vi "Configure lbd for pow meas.vi"(8 "error in (no error)":errorcluster, 10 "Meas lbd (span 0.1 nm)":dbl=895.0 format="%#.6g", 11 "VISA resource name":refnum<visa-resource-name>) -> (0 "error out":errorcluster, 3 "VISA resource name out":refnum<visa-resource-name>)   [LabVIEW 2021, in "Ceyear.lvlib"]
doc: "Configures the frequency range of the spectrum analyzer using the center frequency and the frequency span. If span corresponds to zero Hertz, then the spectrum analyzer operates in time-domain mode. Otherwise, spectrum analyzer operates in frequency-domain mode.\n\n Frequency Start = Center Frequency - Span/2\n Frequency Stop = Center Frequency + Span/2"
uses:
  <instrlib>/Ceyear/Ceyear.lvlib
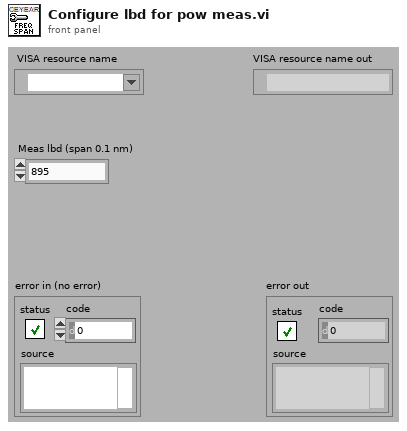
[diagram p1: front panel]
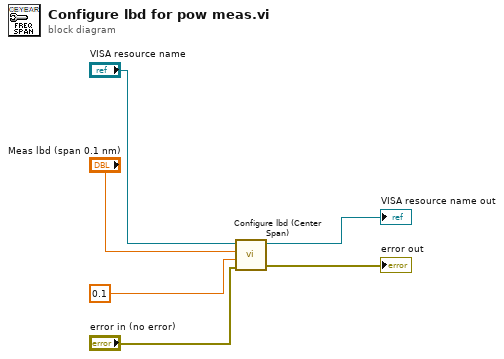
[diagram p0: block diagram]
diagram:
  n1 = call <instrlib>:"Configure lbd (Center Span).vi"("error in (no error)"="error in (no error)", "Span (0.1 - 1100 nm)"=0.1, "Center lbd (600.05 - 1699.95 nm)"="Meas lbd (span 0.1 nm)", "VISA resource name"="VISA resource name") -> ("error out"=→"error out":errorcluster, "VISA resource name out"=→"VISA resource name out":refnum<visa-resource-name>)  [unwired: 6 in]
